vi "Timestamp to ISO8601 String.vi"(5 "Delimiter (system)":T1, 7 "Unit (ms)":T2=enum."millisecond", 9 "UTC? (F)":bool, 11 "Timestamp (now)":timestamp) -> (3 "ISO8601 String":string)   [LabVIEW 2013]
doc: "Converts a <b>Timestamp</b> to <b>ISO8601 String</b>.\n\n<b>UTC?:</b> True: Time in Coordinated Universal Time. False (default): Time in user's local time zone.\n\n<b>Units</b>: Seconds field precision; default is milliseconds."
uses:
  Seconds Units -- enum.ctl
  Locale -- enum.ctl
  Epoch_NotationLocale.vi
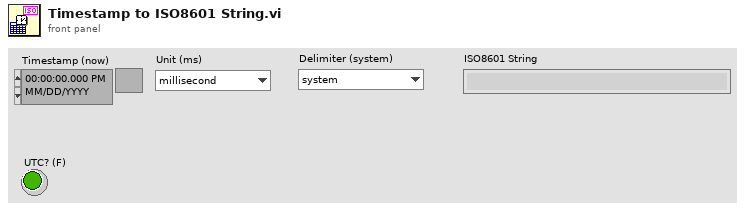
[diagram p1: front panel]
types:
  T1 = typedef "Locale -- enum.ctl" = enum16{"system", "Dot notation", "Comma notation", "custom"}
  T2 = typedef "Seconds Units -- enum.ctl" = enum16{"second", "millisecond", "microsecond", "nanosecond"}
  T3 = typedef "LVDateTimeRec.ctl" = cluster{"fractional second":dbl, "second":i32, "minute":i32, "hour":i32, "day of month":i32, "month":i32, "year":i32, "day of week":i32, "day of year":i32, "DST":i32}
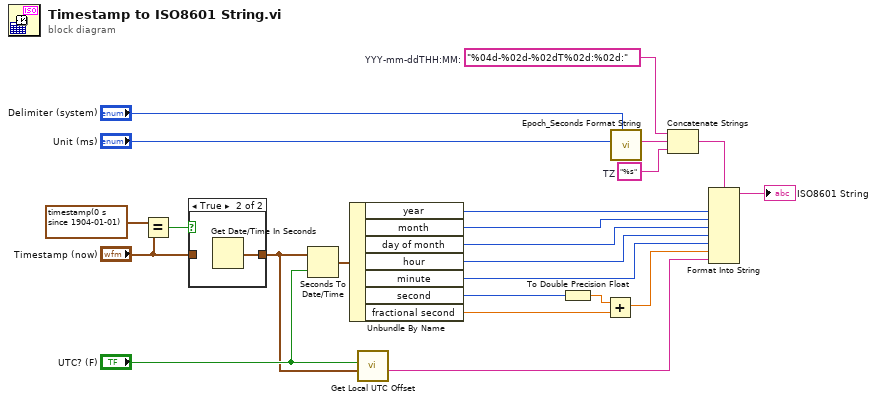
[diagram p0: block diagram]
diagram:
  w5 = "%s"  # TZ
  w6 = "%04d-%02d-%02dT%02d:%02d:"  # YYY-mm-ddTHH:MM:
  n1 = Equal?(x=timestamp(0 s since 1904-01-01), y="Timestamp (now)") -> (x = y?=w13:bool)
  n2 = case shown="True" w13 {
    tunnel: [w24 w25] -> w11
    tunnel: "Timestamp (now)" -> [w24 _]
    frame False {
    }
    frame True {
      n3 = Get Date/Time In Seconds() -> (seconds since 1Jan1904=w25:timestamp)
    }
  }
  n4 = Seconds To Date/Time(time stamp (now)=w11, to UTC (F)="UTC? (F)") -> (date time rec=w21:T3)
  n5 = Unbundle By Name(w21) -> ("year"=w15:i32, "month"=w19:i32, "day of month"=w20:i32, "hour"=w18:i32, "minute"=w17:i32, "second"=w10:i32, "fractional second"=w8:dbl)
  n6 = call "Get Local UTC Offset.vi"("timestamp (now)"=w11, "UTC? (F)"="UTC? (F)") -> ("UTC Offset String"=w16:string)  [unwired: 6 in, 3 out]
  n7 = To Double Precision Float(number=w10) -> (double precision float=w7:dbl)
  n8 = Add(x=w7, y=w8) -> (x+y=w9:dbl)
  n9 = call "Epoch_Seconds Format String.vi"("Delimiter (system)"="Delimiter (system)", "Unit (ms)"="Unit (ms)") -> ("format string"=w3:string)  [unwired: 9 in]
  n10 = Concatenate Strings(w6, w3, w5) -> (w2:string)
  n11 = Format Into String(format string=w2, w15, w19, w20, w18, w17, w9, w16) -> (resulting string=→"ISO8601 String":string)  [unwired: 2 in, 1 out]
